vi "main_scada.vi"() -> ()   [LabVIEW 2015]
uses:
  <vilib>/MakerHub/LINX/Public/Peripherals/Digital/Digital Write 1 Chan.vi
  <vilib>/MakerHub/LINX/Public/Peripherals/Digital/Digital Write N Chans.vi
  <vilib>/MakerHub/LINX/Private/Local IO/LinxDigitalWrite.vi
  <vilib>/MakerHub/LINX/Public/Utilities/Check Channel.vi
  <vilib>/MakerHub/LINX/Public/Utilities/Open Serial.vi
  <vilib>/MakerHub/LINX/Private/Utilties/Generate Error.vi
  <vilib>/MakerHub/LINX/LMH-LINX.lvlib
  <vilib>/MakerHub/LINX/Public/Sensors/Distance/Ultrasonic/Ultrasonic.lvlib
panel:
  out "cm":dbl
  out "Que esta saliendo":dbl
  out "Bajo Nivel":bool
  out "Alto nivel":bool
  out "?":cluster{"SetPoint":dbl, dbl}(graph)={"SetPoint"=0.0, 6.790130396434781}
  out "Slide":dbl(slide) scale=0.0..100.0
  in  "stop":bool
  out "Loop Rate (Hz)":u32
  out "Tiempo de Ejecución":dbl
  out "Error Out":errorcluster
  in  "Channel Alto":u8=6
  in  "Channel Bajo":u8=5
  in  "Alerta N. Alto":dbl=65.0 min=0.0 max=100.0
  in  "Alerta N. Bajo":dbl=20.0 min=0.0 max=100.0
  out "LED Valvula":bool
  out "Meter":dbl(knob) scale=0.0..100.0
  in  "Sensor Ultrasónico":T1={"Canal Trigger (O)"=8, "Canal Echo (I)"=7, "Canal Relay"=9, "Canal Led Valvula"=10}
  in  "SetPoint":dbl=60.0 min=0.0 max=100.0
  in  "Compensacion de altura del sensor":dbl
  in  "Altura del tanque":dbl=20.7
  out "Tank":dbl(slide) scale=0.0..100.0
  in  "Serial Port":refnum<visa-resource-name>="COM3"
  # "cm"
  # "cm"
  # "%"
  # "%"
  # "segundos"
  # "%"
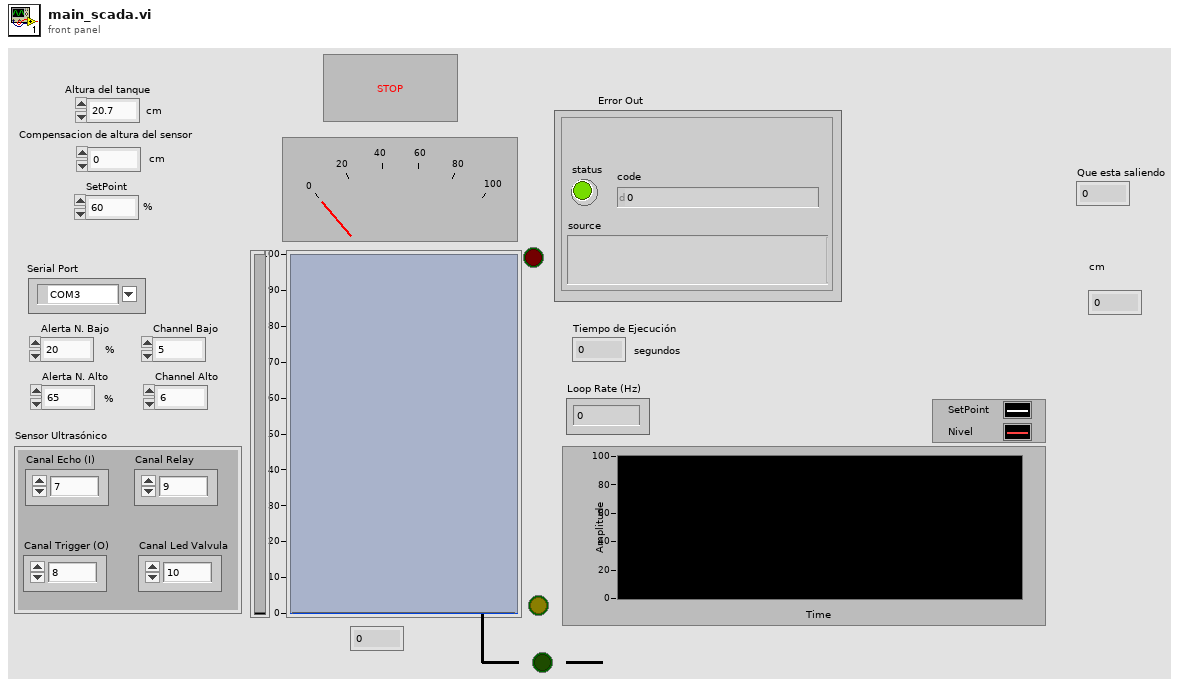
[diagram p1: front panel]
types:
  T1 = cluster{"Canal Trigger (O)":u8, "Canal Echo (I)":u8, "Canal Relay":u8, "Canal Led Valvula":u8}
  T2 = typedef "LMH-LINX.lvlib/LINX Ref.ctl" = cluster{"IO":T3, "Interface":T4, "LINX Device Config":T5}
  T3 = typedef "LMH-LINX.lvlib/Platform.ctl" = enum16{"Remote", "Local"}
  T4 = typedef "LMH-LINX.lvlib/Interface.ctl" = enum16{"Serial", "TCP"}
  T5 = typedef "LMH-LINX.lvlib/Device.lvlib/LINX Device Config.ctl" = cluster{"Interface":T4, "COM Port":refnum<visa-resource-name>, "TCP Configuration":T6, "Device Family":u8, "Device ID":u8, "Device Name":string, "TCP Ref":refnum<k5>, "Channels":T7}
  T6 = typedef "LMH-LINX.lvlib/Device.lvlib/TCP Config.ctl" = cluster{"IP Address":string, "Port":u16}
  T7 = typedef "LMH-LINX.lvlib/Channels.ctl" = cluster{"DI":u8[], "DO":u8[], "AI":u8[], "AO":u8[], "PWM":u8[], "QE":u8[], "UART":u8[], "I2C 2":u8[], "SPI":u8[], "CAN":u8[], "Servo":u8[], "AI Ref (V)":dbl, "AI Resolution (Bits)":u8, "AO Ref (V)":dbl, "AO Resolution (Bits)":u8}
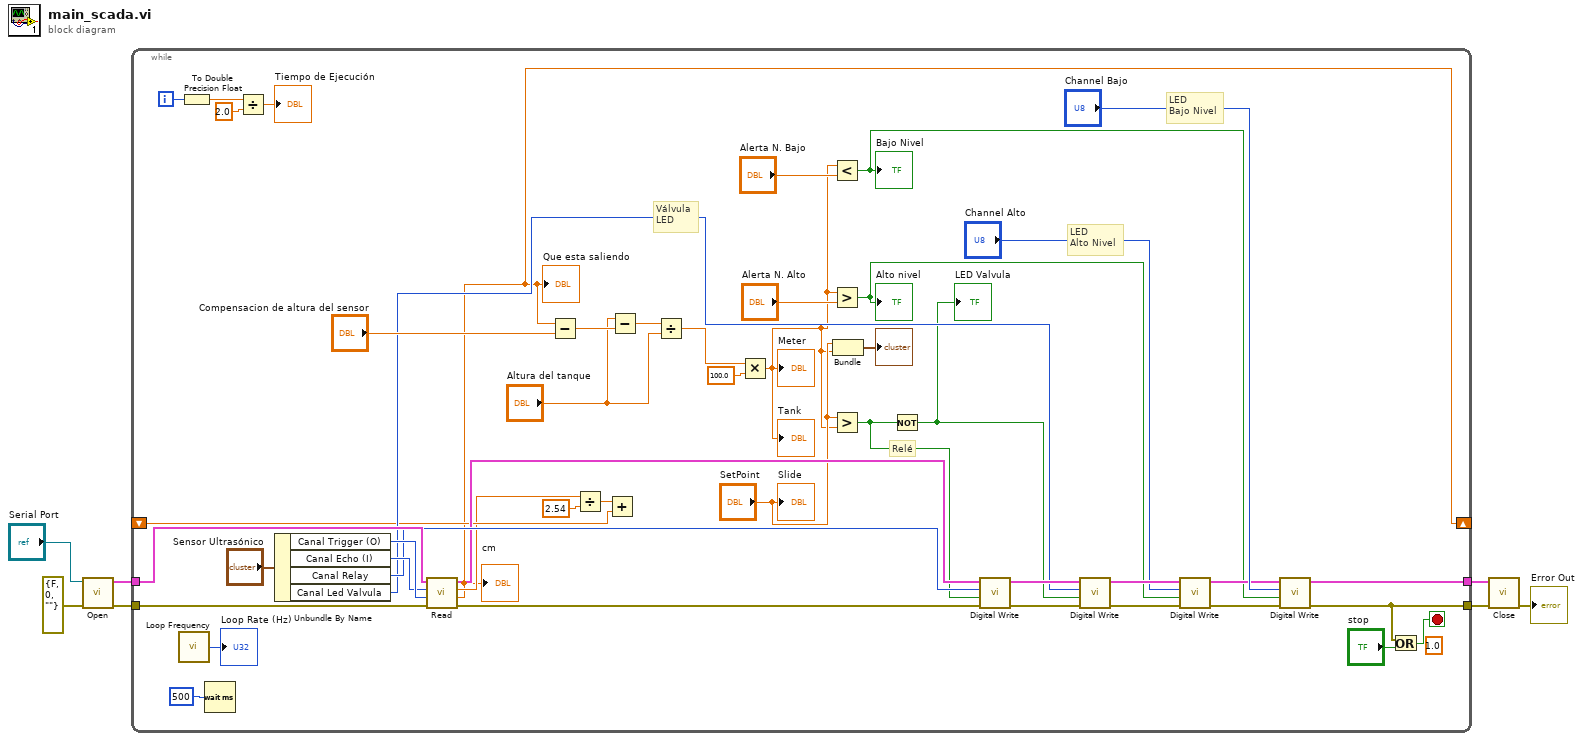
[diagram p0: block diagram]
diagram:
  n1 = call-poly <vilib>:"Open.vi"("Error In"=errorcluster {"status"=FALSE, "code"=0, "source"=""}, "Serial Port"="Serial Port") -> ("Error Out"=w5:errorcluster, "LINX Resource"=w6:T2)  [unwired: 7 in, 1 out]
  n2 = while {
    tunnel: w6 -> [w51]
    tunnel: w5 -> [w50]
    tunnel: [w27] -> w4
    tunnel: [w19] -> w3
    shift-right: [w9] -> _
    shift-left: _ -> [w13]
    i -> [w25]
    stop <- w20 stop-if-true
    (unwired) 1.0 ("y")
    # "LED \nBajo Nivel"
    # "LED \nAlto Nivel"
    # "Válvula \nLED"
    # "Relé"
    n3 = call <vilib>:"Loop Frequency.vi"() -> ("Loop Rate (Hz)"=→"Loop Rate (Hz)":u32)
    n4 = To Double Precision Float(number=w25) -> (double precision float=w22:dbl)
    n5 = Wait (ms)(milliseconds to wait=u32 500) -> ()  [unwired: 1 out]
    n6 = Divide(x=w22, y=2.0) -> (x/y=→"Tiempo de Ejecución":dbl)
    n7 = Unbundle By Name("Sensor Ultrasónico") -> ("Canal Trigger (O)"=w53:u8, "Canal Echo (I)"=w52:u8, "Canal Relay"=w43:u8, "Canal Led Valvula"=w38:u8)
    n8 = call <vilib>:"Read.vi"("Error In"=w50, "DO Channel"=w53, "DI Channel"=w52, "LINX Resource"=w51) -> ("Error Out"=w41:errorcluster, "Centimeters"=w9:dbl, "Inches"=w11:dbl, "LINX Resource"=w42:T2)  [unwired: 4 in]
    "Que esta saliendo" <- w9
    "cm" <- w9
    n9 = Subtract(x=w9, y="Compensacion de altura del sensor") -> (x-y=w48:dbl)
    n10 = Divide(x=w11, y=2.54) -> (x/y=w10:dbl)
    n11 = Add(x=w10, y=w13) -> ()  [unwired: 1 out]
    n12 = Subtract(x="Altura del tanque", y=w48) -> (x-y=w47:dbl)
    n13 = Divide(x=w47, y="Altura del tanque") -> (x/y=w45:dbl)
    n14 = Multiply(x=w45, y=100.0) -> (x*y=w8:dbl)
    "Tank" <- w8
    "Meter" <- w8
    n15 = Less?(x=w8, y="Alerta N. Bajo") -> (x < y?=w14:bool)
    "Bajo Nivel" <- w14
    n16 = Greater?(x=w8, y="Alerta N. Alto") -> (0:w15:bool)
    "Alto nivel" <- w15
    n17 = Greater?(x="SetPoint", y=w8) -> (0:w37:bool)
    n18 = Bundle("SetPoint"="SetPoint", w8) -> (→"?":cluster{"SetPoint":dbl, dbl})  [unwired: 1 in]
    n19 = Not(x=w37) -> (.not. x?=w36:bool)
    "LED Valvula" <- w36
    n20 = call-poly <vilib>:"Digital Write.vi"("Error In"=w41, "Output Value"=w37, "DO Channel"=w43, "LINX Resource"=w42) -> ("Error Out"=w39:errorcluster, "LINX Resource"=w40:T2)  [unwired: 6 in]
    n21 = call-poly <vilib>:"Digital Write.vi"("Error In"=w39, "Output Value"=w36, "DO Channel"=w38, "LINX Resource"=w40) -> ("Error Out"=w32:errorcluster, "LINX Resource"=w33:T2)  [unwired: 6 in]
    n22 = call-poly <vilib>:"Digital Write.vi"("Error In"=w32, "Output Value"=w15, "DO Channel"="Channel Alto", "LINX Resource"=w33) -> ("Error Out"=w28:errorcluster, "LINX Resource"=w29:T2)  [unwired: 6 in]
    n23 = call-poly <vilib>:"Digital Write.vi"("Error In"=w28, "Output Value"=w14, "DO Channel"="Channel Bajo", "LINX Resource"=w29) -> ("Error Out"=w19:errorcluster, "LINX Resource"=w27:T2)  [unwired: 6 in]
    n24 = Or(x=w19, y="stop") -> (x .or. y?=w20:bool)
    "Slide" <- "SetPoint"
  }
  n25 = call <vilib>:"Close.vi"("Error In"=w3, "LINX Resource"=w4) -> ("Error Out"=→"Error Out":errorcluster)  [unwired: 9 in]
